vi "Evaluate Digital Edge Trigger.vi"(8 "error in (no error)":errorcluster, 10 "Trigger Data":dbl[](array[numeric]), 11 "Digital Edge Trigger in":refnum<class "Digital Edge Trigger.lvclass">) -> (0 "error out":errorcluster, 2 "Trigger":bool, 3 "Digital Edge Trigger out":refnum<class "Digital Edge Trigger.lvclass">)   [LabVIEW 2015, in "Digital Edge Trigger.lvclass"]
uses:
  Digital Edge Trigger.lvclass
  Digital Edge Trigger.lvclass/Digital Edge Trigger.ctl
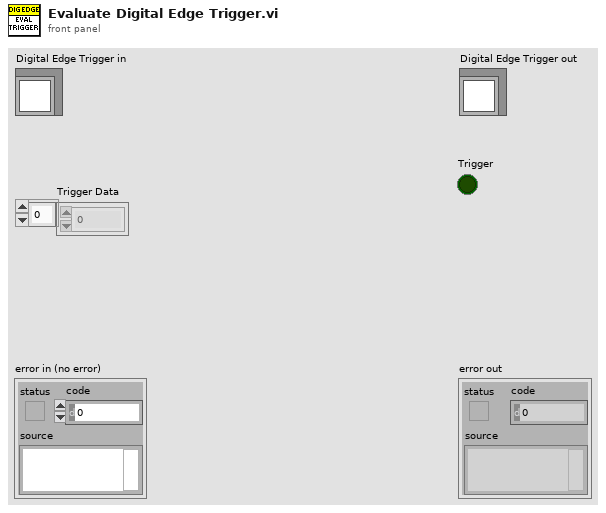
[diagram p1: front panel]
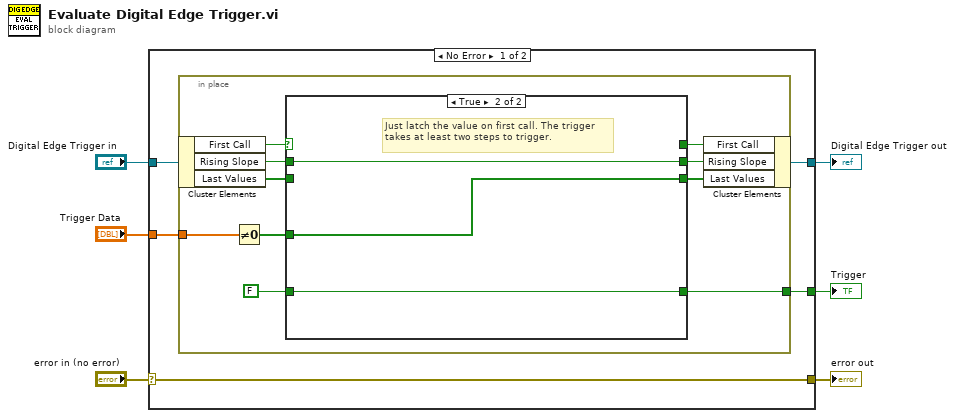
[diagram p0: block diagram]
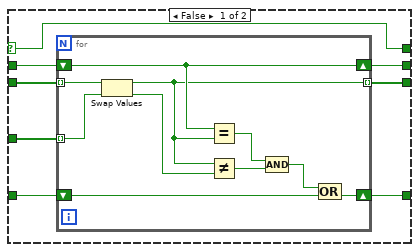
[diagram p2: hidden frame]
diagram:
  n1 = case shown="No Error" "error in (no error)" {
    selector: "error in (no error)" -> [w7 w44]
    tunnel: "Digital Edge Trigger in" -> [w11 w43]
    tunnel: [w10 w43] -> w5
    tunnel: "Trigger Data" -> [w9 _]
    tunnel: [w8 _] -> w3
    tunnel: [w7 w44] -> w1
    frame No Error {
      n2 = in-place {
        in-place-border: w9 -> [w14]
        in-place-border: [w17] -> w8
        n3 = in-place-cluster #1(w11) -> ("First Call"=w16:bool, "Rising Slope"=w21:bool, "Last Values"=w19:bool[])
        n4 = Not Equal To 0?(x=w14) -> (x != 0?=w13:bool[])
        n5 = case shown="True" w16 {
          selector: w16 -> [w24 _]
          tunnel: w21 -> [w27 w42]
          tunnel: [w26 w42] -> w20
          tunnel: w19 -> [w29 _]
          tunnel: [w25 w41] -> w18
          tunnel: [w28 w40] -> w17
          tunnel: [w24 _] -> w15
          tunnel: w13 -> [w23 w41]
          tunnel: FALSE -> [w22 w40]
          frame False {
            n6 = for {
              tunnel: w29 -> [w33] mode=indexing
              shift-right: [w36] -> w26
              shift-left: w27 -> [w36]
              tunnel: [w32] -> w25 mode=indexing
              shift-right: [w35] -> w28
              shift-left: w22 -> [w34]
              tunnel: w23 -> [w30] mode=indexing
              n7 = Swap Values(12:w33, 14:w30) -> (1:w32:bool, 3:w31:bool)  [unwired: 1 in]
              n8 = Equal?(x=w36, y=w32) -> (x = y?=w37:bool)
              n9 = Not Equal?(x=w32, y=w31) -> (x != y?=w38:bool)
              n10 = Compound Arithmetic op=AND(w37, w38) -> (w39:bool)
              n11 = Compound Arithmetic op=OR(w39, w34) -> (w35:bool)
            }
          }
          frame True {
            # "Just latch the value on first call. The trigger takes at least two steps to trigger."
          }
        }
        n12 = in-place-cluster #1("First Call"=w15, "Rising Slope"=w20, "Last Values"=w18) -> (w10:refnum<class "Digital Edge Trigger.lvclass">)
      }
    }
    frame Error {
    }
  }
  "error out" <- w1
  "Digital Edge Trigger out" <- w5
  "Trigger" <- w3
